vi "LogEngine.LogFile.Create.vi"(10 "Port":string, 11 "Project Folder":path) -> (0 "error out":errorcluster, 1 "Continue":bool, 2 "Status":string, 3 "Byte Stream File out":refnum<file>)   [LabVIEW 2025, in "XNET Bus Monitor Client.lvlib"]
uses:
  XNET Bus Monitor Client.lvlib
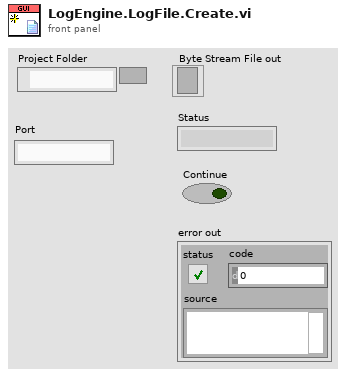
[diagram p1: front panel]
types:
  T1 = enum16{"open", "replace", "create", "open or create", "replace or create", "replace or create with confirmation"}
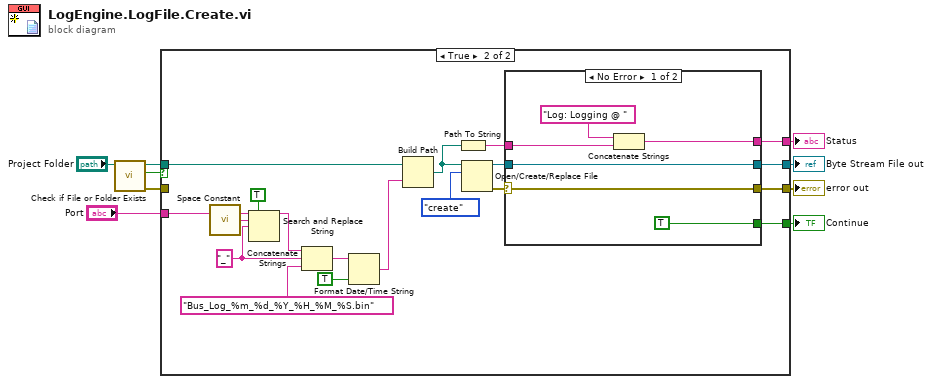
[diagram p0: block diagram]
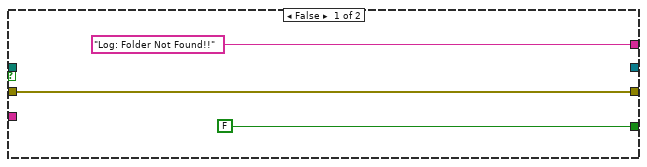
[diagram p2: hidden frame]
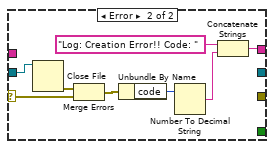
[diagram p3: hidden frame]
diagram:
  n1 = call <vilib>:"Check if File or Folder Exists.vi"("path"="Project Folder") -> ("error out"=w9:errorcluster, "file or folder exists?"=w8:bool, "dup path"=w7:path)  [unwired: 8 in]
  n2 = case shown="True" w8 {
    tunnel: [w11 w30] -> w2
    tunnel: [_ w29] -> w3
    tunnel: [FALSE w27] -> w4
    tunnel: ["Log: Folder Not Found!!" w24] -> w5
    tunnel: w7 -> [_ w15]
    tunnel: w9 -> [w11 _]
    tunnel: "Port" -> [_ w22]
    frame False {
    }
    frame True {
      w18 = "_" ("replace string (\"\")")
      n3 = call <vilib>:"Space Constant.vi"() -> ("String"=w20:string)
      n4 = Search and Replace String(replace all?=TRUE ("replace all? (F)"), input string=w22, search string=w20, replace string=w18) -> (result string=w19:string)  [unwired: 4 in, 3 out]
      n5 = Concatenate Strings(w19, w18, "Bus_Log_%m_%d_%Y_%H_%M_%S.bin" ("time format string (%c)")) -> (w16:string)
      n6 = Format Date/Time String(time format string (%c)=w16, UTC format=TRUE) -> (date/time string=w23:string)  [unwired: 1 in]
      n7 = Build Path(base path=w15, name or relative path=w23) -> (appended path=w14:path)
      n8 = Path To String(path=w14) -> (string=w13:string)
      n9 = Open/Create/Replace File(file path (use dialog)=w14, operation (0:open)=T1."create") -> (refnum out=w31:refnum<file>, error out=w28:errorcluster)  [unwired: 4 in, 1 out]
      n10 = case shown="No Error" w28 {
        selector: w28 -> [w36 w43]
        tunnel: w31 -> [w35 w45]
        tunnel: [w36 _] -> w30
        tunnel: [w35 _] -> w29
        tunnel: [TRUE _] -> w27
        tunnel: [w33 w38] -> w24
        tunnel: w13 -> [w32 _]
        frame No Error {
          n11 = Concatenate Strings("Log: Logging @ " ("string"), w32) -> (w33:string)
        }
        frame Error {
          n12 = Close File(refnum=w45) -> (error out=w44:errorcluster)  [unwired: 1 in, 1 out]
          n13 = Merge Errors(w44, w43) -> (w42:errorcluster)
          n14 = Unbundle By Name(w42) -> ("code"=w41:i32)
          n15 = Number To Decimal String(number=w41) -> (decimal integer string=w40:string)  [unwired: 1 in]
          n16 = Concatenate Strings("Log: Creation Error!! Code: ", w40) -> (w38:string)
        }
      }
    }
  }
  "Status" <- w5
  "Continue" <- w4
  "Byte Stream File out" <- w3
  "error out" <- w2
